vi "SetLayoutInfo.vi"(8 "error in (no error)":errorcluster, 10 "Layout cluster":T1, 11 "Column in":refnum<class "Column.lvclass">) -> (0 "error out":errorcluster, 3 "Column out":refnum<class "Column.lvclass">)   [LabVIEW 2013, in "Column.lvclass"]
doc: "Used by Layout dialog. Only the isDisplayed? element of LayoutCluster is set. To configure colum appearance, use ConfigAppearance.vi (which is utilized by Display Info.vi for each device)."
uses:
  Column.lvclass
  TypeDefs/ColumnLayoutCluster.ctl
  Column.lvclass/Column.ctl
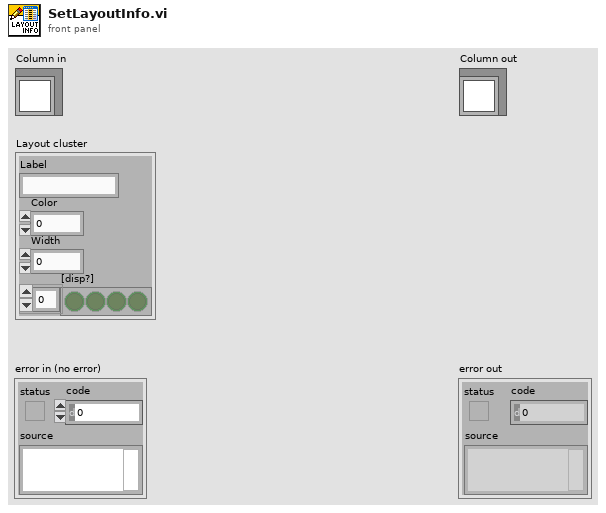
[diagram p1: front panel]
types:
  T1 = typedef "ColumnLayoutCluster.ctl" = cluster{"Label":string, "Color":u32, "Width":u32, "[disp?]":bool[]}
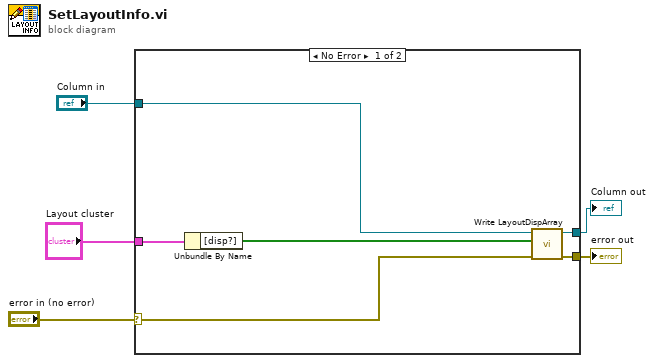
[diagram p0: block diagram]
diagram:
  n1 = case shown="No Error" "error in (no error)" {
    selector: "error in (no error)" -> [w9 w13]
    tunnel: [w10 w13] -> w3
    tunnel: [w11 w12] -> w2
    tunnel: "Column in" -> [w7 w12]
    tunnel: "Layout cluster" -> [w8 _]
    frame No Error {
      n2 = Unbundle By Name(w8) -> ("[disp?]"=w6:bool[])
      n3 = call "Write LayoutDispArray.vi"("error in (no error)"=w9, "Layout disp? array"=w6, "Column in"=w7) -> ("error out"=w10:errorcluster, "Column out"=w11:refnum<class "Column.lvclass">)  [unwired: 7 in]
    }
    frame Error {
    }
  }
  "error out" <- w3
  "Column out" <- w2
